vi "RichToFlatrouteguide_Feature.vi"(5 "OutputClusterType":T1, 11 "InputCluster":T3) -> (3 "OutputCluster":T1)   [LabVIEW 2019, in "route_guide_client.lvlib"]
uses:
  route_guide_client.lvlib
  routeguide_Feature.ctl
  routeguide_Point.ctl
  routeguide_Feature_Flat.ctl
  routeguide_Point_Flat.ctl
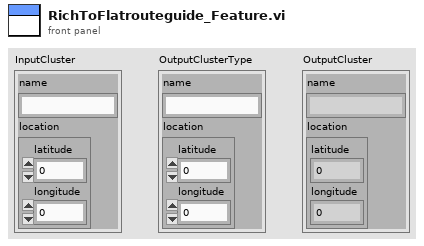
[diagram p1: front panel]
types:
  T1 = typedef "route_guide_client.lvlib/routeguide_Feature_Flat.ctl" = cluster{"name":string, "location":T2}
  T2 = typedef "route_guide_client.lvlib/routeguide_Point_Flat.ctl" = cluster{"latitude":i32, "longitude":i32}
  T3 = typedef "route_guide_client.lvlib/routeguide_Feature.ctl" = cluster{"name":string, "location":T4}
  T4 = typedef "route_guide_client.lvlib/routeguide_Point.ctl" = cluster{"latitude":i32, "longitude":i32}
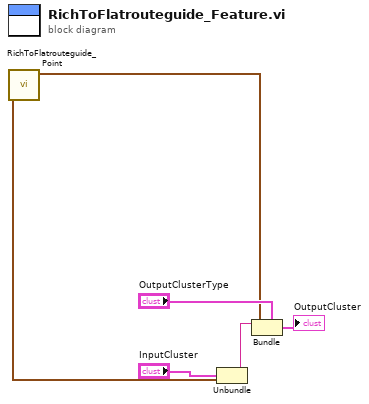
[diagram p0: block diagram]
diagram:
  n1 = Unbundle "Unbundle"("InputCluster") -> ("name"=w3:string, "location"=w2:T4)
  n2 = call "RichToFlatrouteguide_Point.vi"("InputCluster"=w2) -> ("OutputCluster"=w1:T2)  [unwired: 10 in]
  n3 = Bundle "Bundle"(cluster="OutputClusterType", "name"=w3, "location"=w1) -> (→"OutputCluster":T1)
